vi "Dictionary.Add Time Values.vi"(8 "error in (no error)":errorcluster, 10 "Data (Dictionary)":T1[](array[typedef])) -> (0 "error out":errorcluster, 2 "Dictionary":T1[](array[typedef]))   [LabVIEW 2019, in "Conversion.lvclass"]
uses:
  Conversion.lvclass
  Data/Typedefs/Dictionary--cluster.ctl
  Data/Data.lvclass
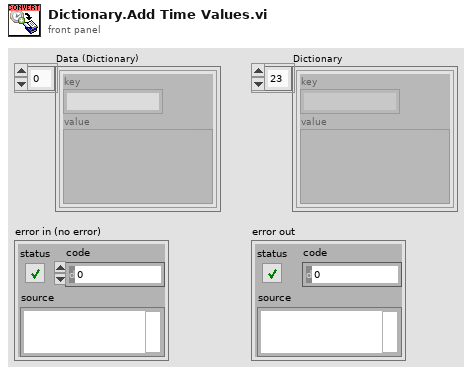
[diagram p1: front panel]
types:
  T1 = typedef "Data.lvclass/Dictionary--cluster.ctl" = cluster{"key":string, "value":variant}
  T2 = typedef "Dictionary Object RefNum__ogtk.ctl" = refnum<k1>
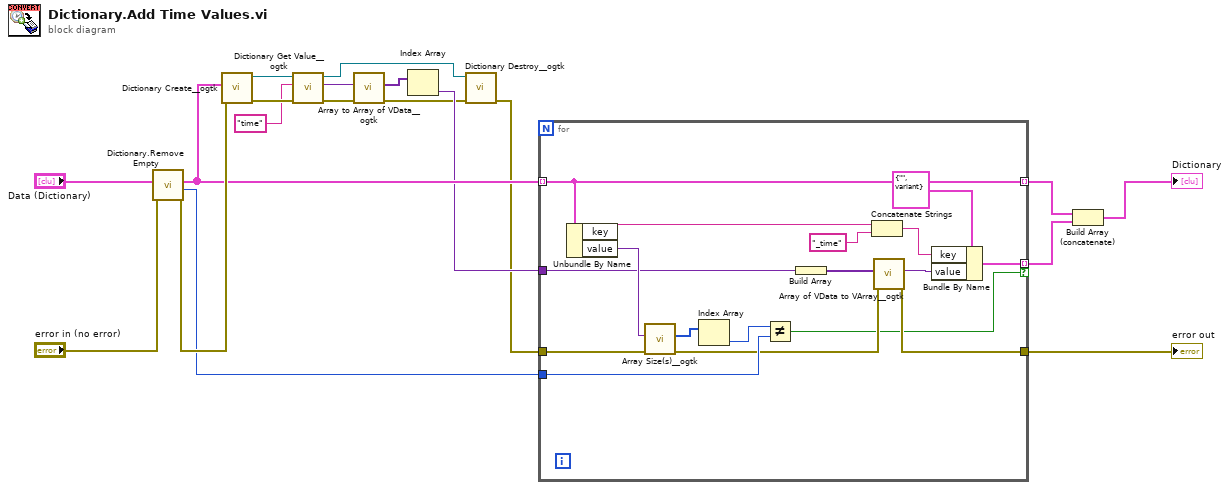
[diagram p0: block diagram]
diagram:
  n1 = call "Dictionary.Remove Empty.vi"("error in (no error)"="error in (no error)", "Data (Dictionary)"="Data (Dictionary)") -> ("error out"=w11:errorcluster, "max Array Size"=w8:i32, "Data (Dictionary)"=w10:T1[])  [unwired: 7 in]
  n2 = call "Dictionary Create__ogtk.vi"("error in (no error)"=w11, "initial dictionary (empty)"=w10) -> ("error out"=w18:errorcluster, "dictionary out"=w17:T2)  [unwired: 8 in]
  n3 = call "Dictionary Get Value__ogtk.vi"("error in"=w18, "key"="time", "dictionary"=w17) -> ("error out"=w15:errorcluster, "value"=w14:variant, "dictionary out"=w3:T2)  [unwired: 5 in, 1 out]
  n4 = call "Array to Array of VData__ogtk.vi"("error in (no error)"=w15, "MultiD Array"=w14) -> ("error out"=w2:errorcluster, "1D Array of Variants"=w13:variant[])  [unwired: 8 in]
  n5 = Index Array(array=w13) -> (element=w4:variant)  [unwired: 1 in]
  n6 = call "Dictionary Destroy__ogtk.vi"("error in (no error)"=w2, "dictionary"=w3) -> ("error out"=w1:errorcluster)  [unwired: 9 in]
  n7 = for {
    tunnel: w8 -> [w35]
    tunnel: w10 -> [w24] mode=indexing
    tunnel: [w24] -> w6 mode=indexing
    tunnel: w1 -> [w36]
    tunnel: [w27] -> w19
    tunnel: [w30] -> w7 mode=indexing if=w26
    tunnel: w4 -> [w22]
    n8 = Unbundle By Name(w24) -> ("key"=w21:string, "value"=w31:variant)
    n9 = call "Array Size(s)__ogtk.vi"("error in (no error)"=w36, "Array"=w31) -> ("error out"=w28:errorcluster, "Size(s)"=w33:u32[])  [unwired: 7 in, 1 out]
    n10 = Index Array(array=w33) -> (element=w32:u32)  [unwired: 1 in]
    n11 = Not Equal?(x=w32, y=w35) -> (x != y?=w26:bool)
    n12 = Build Array(w22) -> (w23:variant[])
    n13 = Concatenate Strings(w21, "_time") -> (w25:string)
    n14 = call "Array of VData to VArray__ogtk.vi"("error in (no error)"=w28, "1D Array of VData"=w23) -> ("error out"=w27:errorcluster, "VArray"=w29:variant)  [unwired: 8 in]
    n15 = Bundle By Name(cluster=T1 {"key"="", "value"=variant} ("key-value"), "key"=w25, "value"=w29) -> (w30:T1)
  }
  "error out" <- w19
  n16 = Build Array (concatenate)(w6, w7) -> (→"Dictionary":T1[])
